vi "Autodiscover Group Async.vi"(10 "Discovery":T5, 11 "RemoteDataService in":refnum<class "RemoteDataService.lvclass">) -> ()   [LabVIEW 2020, in "Vecto.lvlib" / "RemoteDataService.lvclass"]
uses:
  RemoteDataService.lvclass
  lv-volatus/messages/Discovery/Data.ctl
  lv-volatus/messages/Service/Data.ctl
  lv-volatus/messages/ServiceType/Enumeration.ctl
  Publish Config Response.ctl
  Publish Config Response Group.ctl
  Publish Config.ctl
  Group Data Type.ctl
  RemoteDataService.lvclass/RemoteDataService.ctl
  Group Info.ctl
  Channel Init.ctl
  d6d46936-9d17-4774-a8db-78bb1b9f4e95.vi
  <vilib>/JDP Science/JSONtext/JSON text to Variant.vi
  ChannelService/Create Group Abstract.vi
  <vilib>/JDP Science/JSONtext/LVClass Serializer/JSONtext LVClass Serializer.lvclass
  Group/Group.lvclass
  Vecto.lvlib
  lv-volatus/messages/ServiceType/ServiceType.lvlib
  <vilib>/httpClient/LabVIEWHTTPClient.lvlib
  VectoConfig/VectoConfig.lvlib
  Group Config/Group Config.lvclass
  ChannelService/ChannelService.lvclass
  lv-volatus/messages/Service/Service.lvlib
  lv-volatus/messages/Discovery/Discovery.lvlib
panel:
  out "Publish Config Response":T1
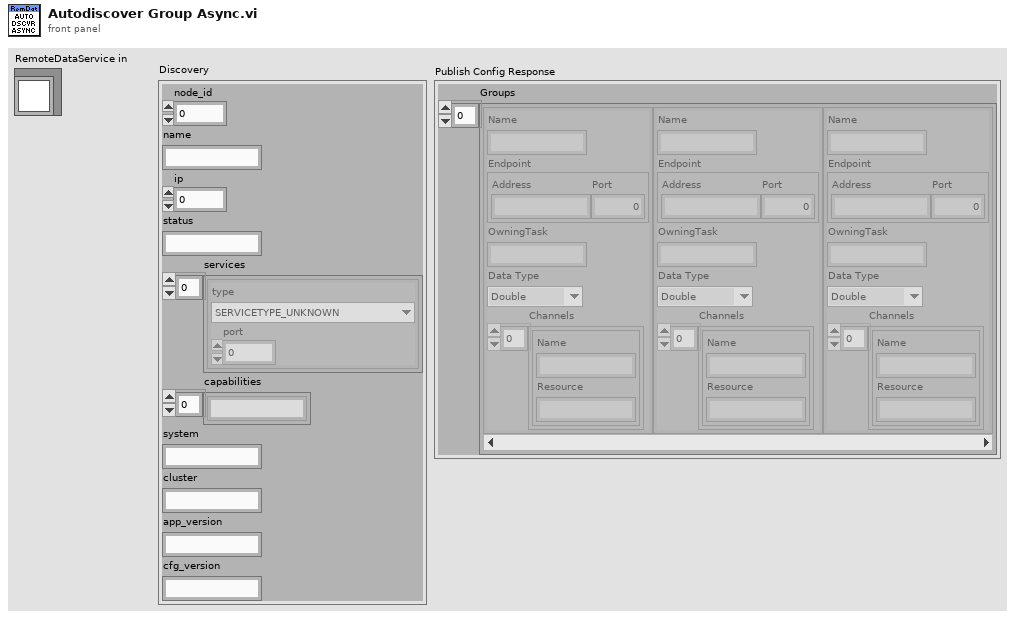
[diagram p1: front panel]
types:
  T1 = typedef "Vecto.lvlib/Publish Config Response.ctl" = cluster{"Groups":T2[]}
  T2 = typedef "Vecto.lvlib/Publish Config Response Group.ctl" = cluster{"Name":string, "Endpoint":T3, "OwningTask":string, "Data Type":T4, "Channels":cluster{"Name":string, "Resource":string}[]}
  T3 = typedef "VectoConfig.lvlib/Publish Config.ctl" = cluster{"Address":string, "Port":u16}
  T4 = typedef "VectoConfig.lvlib/Group Data Type.ctl" = enum16{"Double", "String", "Bool"}
  T5 = typedef "Discovery.lvlib/Data.ctl" = cluster{"node_id":u32, "name":string, "ip":u32, "status":string, "services":T6[], "capabilities":string[], "system":string, "cluster":string, "app_version":string, "cfg_version":string}
  T6 = typedef "Service.lvlib/Data.ctl" = cluster{"type":T7, "port":i32}
  T7 = typedef "ServiceType.lvlib/Enumeration.ctl" = enum16{"SERVICETYPE_UNKNOWN", "SERVICETYPE_TCPSERVER", "SERVICETYPE_HTTPSERVER"}
  T8 = typedef "VectoConfig.lvlib/Group Info.ctl" = cluster{"System":string, "Cluster":string, "Node":string, "Task":string, "Name":string}
  T9 = typedef "VectoConfig.lvlib/Channel Init.ctl" = cluster{"Name":string, "Resource":string, "Unit String":string}
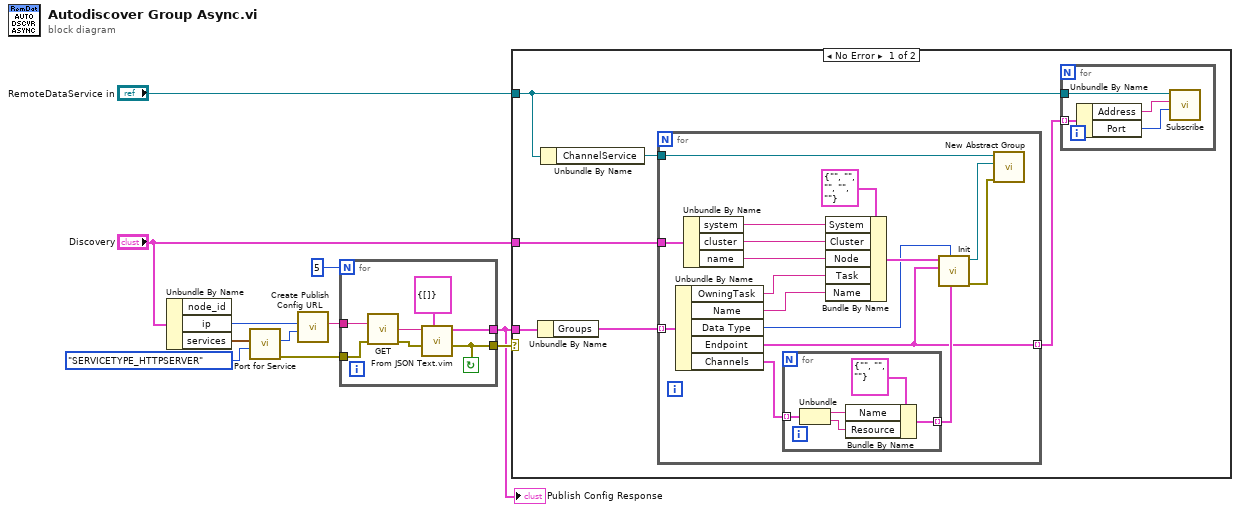
[diagram p0: block diagram]
diagram:
  n1 = Unbundle By Name("Discovery") -> ("ip"=w9:u32, "services"=w11:T6[])  [unwired: 1 out]
  n2 = call "Port for Service.vi"("type"=Enumeration."SERVICETYPE_HTTPSERVER", "services"=w11) -> ("error out"=w6:errorcluster, "port"=w8:i32)  [unwired: 8 in]
  n3 = call "Create Publish Config URL.vi"("port"=w8, "ip"=w9) -> ("String"=w7:string)  [unwired: 9 in]
  n4 = for {
    N: 5 -> [_]
    tunnel: w7 -> [w18]
    tunnel: w6 -> [w17]
    tunnel: [w15] -> w1
    tunnel: [w13] -> w4
    stop <- w13 continue-if-true
    n5 = call <vilib>:"GET.vi"("url"=w18, "error in (no error)"=w17) -> ("body"=w16:string, "error out"=w14:errorcluster)  [unwired: 10 in, 2 out]
    n6 = call "From JSON Text.vim"("Data Type and Default Value"=T1 {"Groups"=[]} ("Publish Config Response"), "error in (no error)"=w14, "JSON"=w16) -> ("error out"=w13:errorcluster, "Data out"=w15:T1)  [unwired: 7 in]
  }
  "Publish Config Response" <- w1
  n7 = case shown="No Error" w4 {
    tunnel: w1 -> [w24 _]
    tunnel: "RemoteDataService in" -> [w20 _]
    tunnel: "Discovery" -> [w21 _]
    frame No Error {
      n8 = Unbundle By Name(w24) -> ("Groups"=w23:T2[])
      n9 = Unbundle By Name(w20) -> ("ChannelService"=w22:refnum<class "ChannelService.lvclass">)
      n10 = for {
        tunnel: w23 -> [w44] mode=indexing
        tunnel: w22 -> [w33]
        tunnel: w21 -> [w42]
        tunnel: [w30] -> w19 mode=indexing
        n11 = Unbundle By Name(w44) -> ("OwningTask"=w37:string, "Name"=w36:string, "Data Type"=w29:T4, "Endpoint"=w30:T3, "Channels"=w35:cluster{"Name":string, "Resource":string}[])
        n12 = Unbundle By Name(w42) -> ("system"=w40:string, "cluster"=w39:string, "name"=w38:string)
        n13 = for {
          tunnel: w35 -> [w47] mode=indexing
          tunnel: [w48] -> w34 mode=indexing
          n14 = Unbundle(w47) -> ("Name"=w46:string, "Resource"=w45:string)
          n15 = Bundle By Name(cluster=T9 {"Name"="", "Resource"="", "Unit String"=""} ("Channel Init"), "Name"=w46, "Resource"=w45) -> (w48:T9)
        }
        n16 = Bundle By Name(cluster=T8 {"System"="", "Cluster"="", "Node"="", "Task"="", "Name"=""} ("Group Info"), "System"=w40, "Cluster"=w39, "Node"=w38, "Task"=w37, "Name"=w36) -> (w41:T8)
        n17 = call "Init.vi"("Channels"=w34, "Group Data Type"=w29, "Multicast Endpoint (None)"=w30, "Group Info"=w41) -> ("error out"=w31:errorcluster, "Group Config out"=w32:refnum<class "Group Config.lvclass">)  [unwired: 6 in]
        n18 = call "New Abstract Group.vi"("error in (no error)"=w31, "Group Config"=w32, "ChannelService in"=w33) -> ()  [unwired: 6 in, 3 out]
      }
      n19 = for {
        tunnel: w20 -> [w28]
        tunnel: w19 -> [w27] mode=indexing
        n20 = Unbundle By Name(w27) -> ("Address"=w26:string, "Port"=w25:u16)
        n21 = call "Subscribe.vi"("Multicast Port"=w25, "Multicast Address"=w26, "RemoteDataService in"=w28) -> ()  [unwired: 7 in, 2 out]
      }
    }
    frame Error {
    }
  }
